vi "InterpolateWave.vi"(8 "输出波形预设":dbl[][](array[numeric])) -> (1 "XY Graph":cluster{"xi used":dbl[], "yi":dbl[]}(graph), 2 "插值后输出波形时间":dbl[](array[numeric]) format="%_6g", 3 "插值后输出波形幅值":dbl[](array[numeric]))   [LabVIEW 2018]
uses:
  <vilib>/gmath/NI_Gmath.lvlib
panel:
  # "第一列代表时间，第二列代表幅值"
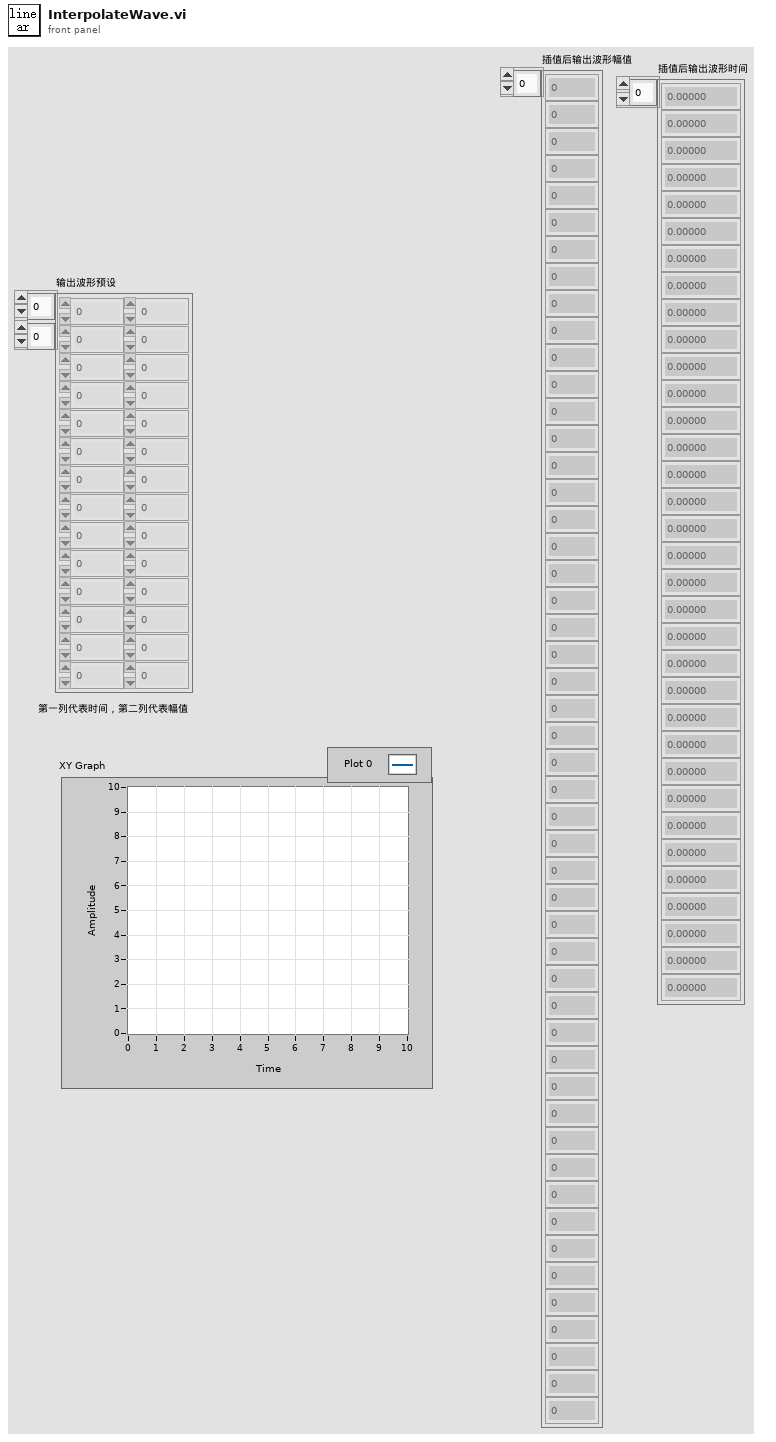
[diagram p1: front panel]
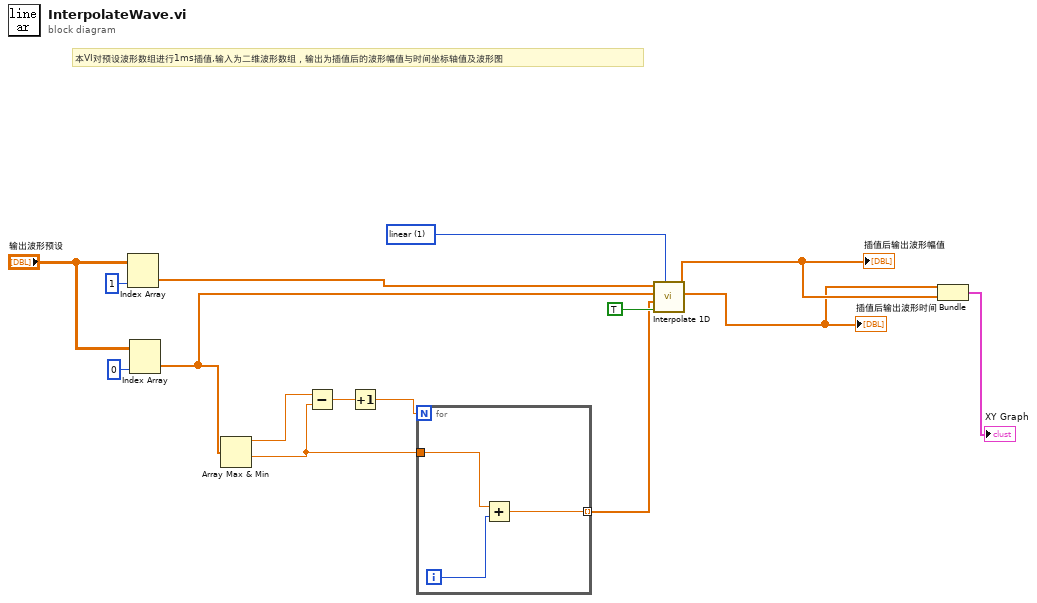
[diagram p0: block diagram]
diagram:
  w15 = 1 items=["nearest", "linear", "spline", "cubic Hermite", "Lagrange"] ("method")
  # "本VI对预设波形数组进行1ms插值,输入为二维波形数组，输出为插值后的波形幅值与时间坐标轴值及波形图"
  n1 = Index Array(array="输出波形预设", index (col)=1 ("disabled index (col)")) -> (element=w11:dbl[])  [unwired: 1 in]
  n2 = Index Array(array="输出波形预设", index (col)=0 ("disabled index (col)")) -> (element=w6:dbl[])  [unwired: 1 in]
  n3 = Array Max & Min(array=w6) -> (max value=w9:dbl, min value=w8:dbl)  [unwired: 2 out]
  n4 = Subtract(x=w9, y=w8) -> (x-y=w4:dbl)
  n5 = Increment(x=w4) -> (x+1=w3:dbl)
  n6 = for {
    N: w3 -> [_]
    tunnel: w8 -> [w17]
    tunnel: [w16] -> w7 mode=indexing
    i -> [w18]
    n7 = Add(x=w17, y=w18) -> (x+y=w16:dbl)
  }
  n8 = call <vilib>:"Interpolate 1D.vi"("method"=w15, "X is monotonic"=TRUE, "xi"=w7, "X"=w6, "Y"=w11) -> ("xi used"=w2:dbl[], "yi"=w5:dbl[])  [unwired: 4 in, 1 out]
  "插值后输出波形幅值" <- w5
  "插值后输出波形时间" <- w2
  n9 = Bundle("xi used"=w2, "yi"=w5) -> (→"XY Graph":cluster{"xi used":dbl[], "yi":dbl[]})  [unwired: 1 in]
